vi "GLdrv_TRIG_COND_COMB.vi"(0 "Connection ID":T2, 5 "COND":i32=1 min=0 max=1, 7 "Combination":T1(ring), 11 "error in (no error)":errorcluster, 13 "Query(f)":bool) -> (4 "Connection ID Out":T2, 8 "Combination out":T1(ring), 15 "error out":errorcluster)   [LabVIEW 2017, in "GL860_Driver.lvlib"]
doc: "各入力CHのトリガをAND検知かOR検知するか設定します\n入力レベルをエッジ検知するかレベル検知するか設定します\nLEVEL：　HIに設定した場合、設定値より上に信号があるときトリガ\nが発生します。LOに設定した場合、設定値より下に信号があるときト\nリガが発生します\nEDGE：　HI（立ち上がり）に設定した場合は、設定値を下から上に突\nき抜けたときにトリガが発生します。LO（立下り）に設定した場合は、\n設定値を上から下に突き抜けたときにトリガが発生します\nOR：　どれか１つのトリガが発生するとトリガが成立します\nAND：　すべてのトリガが同時に発生するとトリガが成立します\n例）　:TRIG:COND0:COMB EDGE,AND (トリガスタートをAND検知でエ\nッジ検出に設定します)\n例）　:TRIG:COND1:COMB LEVEL,OR (トリガストップとOR検知でレベ\nル検出に設定します)"
uses:
  GL860_Driver.lvlib
  ConnectionID.ctl
  GLdrv_RW.ctl
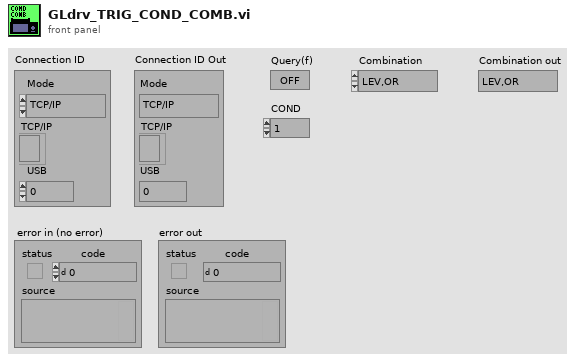
[diagram p1: front panel]
types:
  T1 = enum16{"LEV,OR", "LEV,AND", "EDGE,OR", "EDGE,AND"}
  T2 = typedef "ConnectionID.ctl" = cluster{"Mode":enum16{"TCP/IP", "USB"}, "TCP/IP":refnum<k5>, "USB":i32}
  T3 = typedef "GLdrv_RW.ctl" = enum16{"Auto", "Read", "Write", "Buffer"}
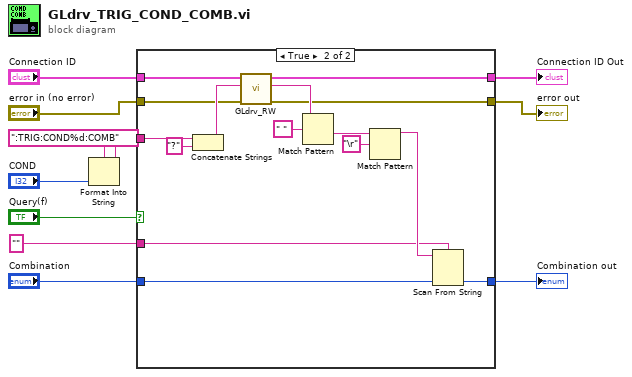
[diagram p0: block diagram]
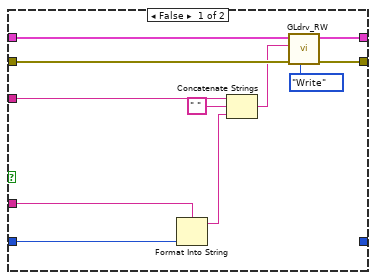
[diagram p2: hidden frame]
diagram:
  n1 = Format Into String(format string=":TRIG:COND%d:COMB" ("Command"), "COND") -> (resulting string=w5:string)  [unwired: 2 in, 1 out]
  n2 = case shown="TRUE" "Query(f)" {
    tunnel: w5 -> [w22 w34]
    tunnel: [w17 w26] -> w11
    tunnel: [w19 w30] -> w10
    tunnel: "Connection ID" -> [w20 w31]
    tunnel: "error in (no error)" -> [w18 w27]
    tunnel: "Combination" -> [w13 w25]
    tunnel: [_ w24] -> w2
    tunnel: "" ("Param") -> [w12 w23]
    frame False {
      n3 = Format Into String(format string=w12, w13) -> (resulting string=w14:string)  [unwired: 2 in, 1 out]
      n4 = Concatenate Strings(w22, " " ("string"), w14) -> (w16:string)
      n5 = call "GLdrv_RW.vi"("Mode(read)"=GLdrv_RW."Write", "error in (no error)"=w18, "data in"=w16, "Connection ID"=w20) -> ("error out"=w17:errorcluster, "Connection ID Out"=w19:T2)  [unwired: 3 in, 3 out]
    }
    frame True {
      n6 = Concatenate Strings(w34, "?" ("string")) -> (w29:string)
      n7 = call "GLdrv_RW.vi"("error in (no error)"=w27, "data in"=w29, "Connection ID"=w31) -> ("error out"=w26:errorcluster, "data out"=w28:string, "Connection ID Out"=w30:T2)  [unwired: 4 in, 2 out]
      n8 = Match Pattern(string=w28, regular expression=" " ("search string/char (-)")) -> (after substring=w35:string)  [unwired: 4 out]
      n9 = Match Pattern(string=w35, regular expression="\r") -> (before substring=w32:string)  [unwired: 4 out]
      n10 = Scan From String(format string=w23, input string=w32, default 1=w25) -> (output 1=w24:T1)  [unwired: 2 in, 3 out]
    }
  }
  "Connection ID Out" <- w10
  "error out" <- w11
  "Combination out" <- w2
